vi "删除.vi"(8 "error in (no error)":errorcluster caption="错误输入（无错误）", 11 "程序 输入":refnum<class "程序.lvclass">) -> (0 "error out":errorcluster caption="错误输出", 3 "程序 输出":refnum<class "程序.lvclass">)   [LabVIEW 2020, in "程序.lvclass"]
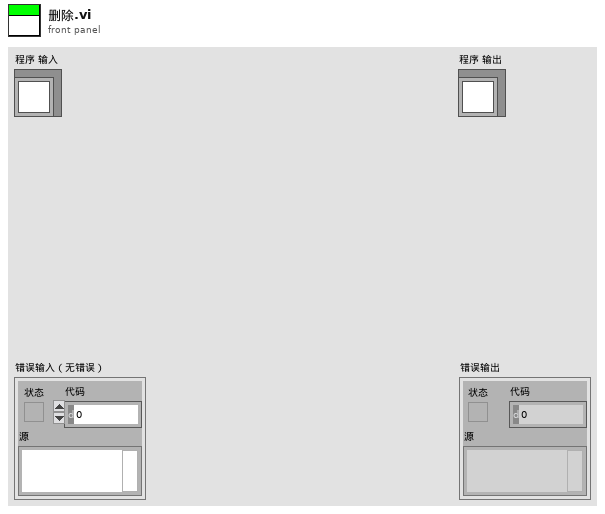
[diagram p1: front panel]
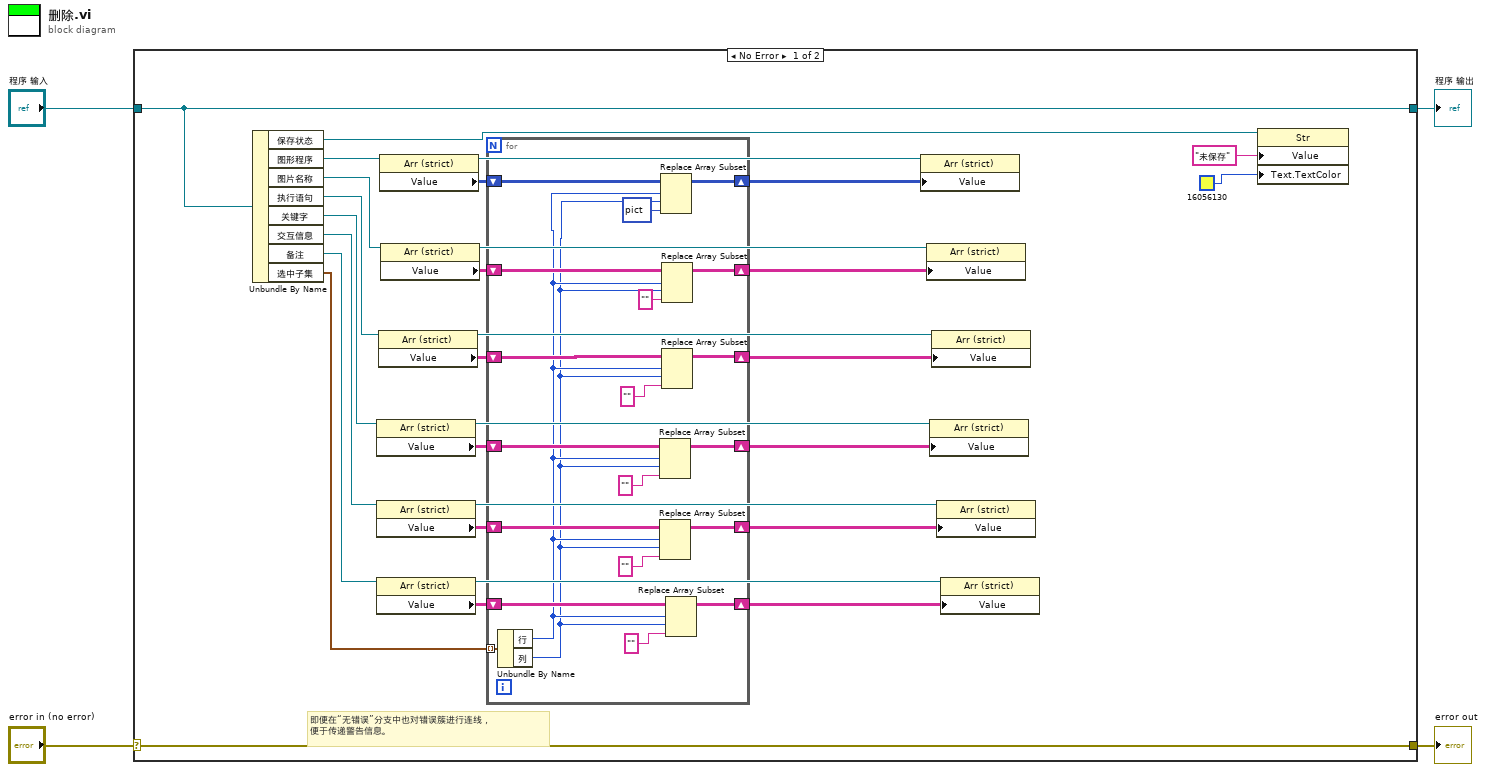
[diagram p0: block diagram]
diagram:
  n1 = case shown="No Error" "error in (no error)" {
    selector: "error in (no error)" -> [w34 w57]
    tunnel: [w34 w57] -> w3
    tunnel: [w20 w56] -> w1
    tunnel: "程序 输入" -> [w20 w56]
    frame No Error {
      # "即便在“无错误”分支中也对错误簇进行连线，\n便于传递警告信息。"
      n2 = Unbundle By Name(w20) -> ("保存状态"=w5:refnum<vi>, "图形程序"=w33:refnum<vi>, "图片名称"=w32:refnum<vi>, "执行语句"=w31:refnum<vi>, "关键字"=w16:refnum<vi>, "交互信息"=w14:refnum<vi>, "备注"=w11:refnum<vi>, "选中子集"=w30:cluster{"行":i32, "列":i32}[])
      n3 = property class="Arr (strict)"(reference=w16) -> (reference out=w17:refnum<vi>, "Value"=w18:string[][])  [unwired: 1 in, 1 out]
      n4 = property class="Arr (strict)"(reference=w14) -> (reference out=w13:refnum<vi>, "Value"=w15:string[][])  [unwired: 1 in, 1 out]
      n5 = property class="Arr (strict)"(reference=w11) -> (reference out=w8:refnum<vi>, "Value"=w10:string[][])  [unwired: 1 in, 1 out]
      n6 = property class="Arr (strict)"(reference=w31) -> (reference out=w27:refnum<vi>, "Value"=w24:string[][])  [unwired: 1 in, 1 out]
      n7 = property class="Arr (strict)"(reference=w33) -> (reference out=w29:refnum<vi>, "Value"=w26:picture[][])  [unwired: 1 in, 1 out]
      n8 = property class="Arr (strict)"(reference=w32) -> (reference out=w28:refnum<vi>, "Value"=w25:string[][])  [unwired: 1 in, 1 out]
      n9 = for {
        tunnel: w30 -> [w55] mode=indexing
        shift-right: [w49] -> w23
        shift-left: w26 -> [w54]
        shift-right: [w47] -> w22
        shift-left: w25 -> [w53]
        shift-right: [w48] -> w21
        shift-left: w24 -> [w50]
        shift-right: [w45] -> w19
        shift-left: w18 -> [w44]
        shift-right: [w40] -> w12
        shift-left: w15 -> [w41]
        shift-right: [w38] -> w9
        shift-left: w10 -> [w37]
        n10 = Unbundle By Name(w55) -> ("行"=w36:i32, "列"=w35:i32)
        n11 = Replace Array Subset(array=w44, new element="" ("新元素/子数组"), index (row)=w36, index (col)=w35) -> (w45:string[][])
        n12 = Replace Array Subset(array=w41, new element="" ("新元素/子数组"), index (row)=w36, index (col)=w35) -> (w40:string[][])
        n13 = Replace Array Subset(array=w54, new element=picture data[5B] ("新元素/子数组"), index (row)=w36, index (col)=w35) -> (w49:picture[][])
        n14 = Replace Array Subset(array=w53, new element="" ("新元素/子数组"), index (row)=w36, index (col)=w35) -> (w47:string[][])
        n15 = Replace Array Subset(array=w50, new element="" ("新元素/子数组"), index (row)=w36, index (col)=w35) -> (w48:string[][])
        n16 = Replace Array Subset(array=w37, new element="" ("新元素/子数组"), index (row)=w36, index (col)=w35) -> (w38:string[][])
      }
      n17 = property class="Arr (strict)"(reference=w29, "Value"=w23) -> ()  [unwired: 1 in, 2 out]
      n18 = property class="Arr (strict)"(reference=w28, "Value"=w22) -> ()  [unwired: 1 in, 2 out]
      n19 = property class="Arr (strict)"(reference=w17, "Value"=w19) -> ()  [unwired: 1 in, 2 out]
      n20 = property class="Arr (strict)"(reference=w27, "Value"=w21) -> ()  [unwired: 1 in, 2 out]
      n21 = property class="Arr (strict)"(reference=w13, "Value"=w12) -> ()  [unwired: 1 in, 2 out]
      n22 = property class="Arr (strict)"(reference=w8, "Value"=w9) -> ()  [unwired: 1 in, 2 out]
      n23 = property class="Str"(reference=w5, "Value"="未保存" ("值"), "Text.TextColor"=u32 16056130) -> ()  [unwired: 1 in, 2 out]
    }
    frame Error {
    }
  }
  "error out" <- w3
  "程序 输出" <- w1
